vi "Process Workflow Range.vi"(8 "Parts":map{string, cluster{"Min":i64, "Max":i64}}(c390), 9 "Current Workflow":string="in", 10 "Workflow Map":map{string, string[]}(c390), 11 "Count In":i64) -> (3 "Count Out":i64)   [LabVIEW 2021]
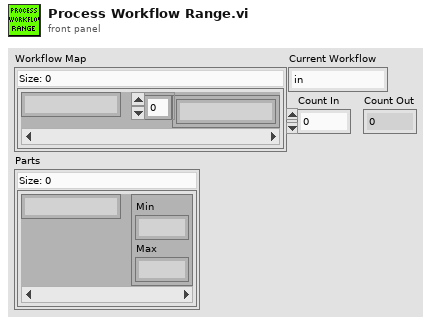
[diagram p1: front panel]
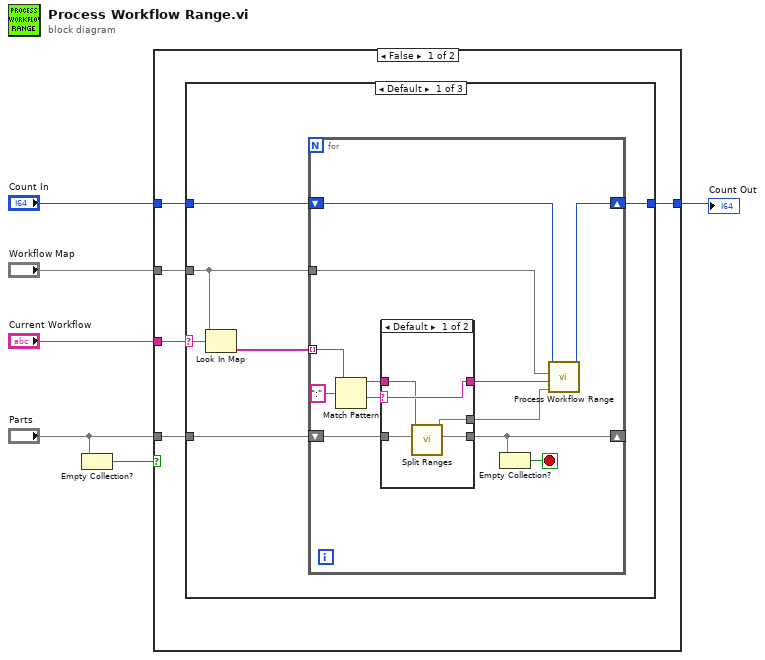
[diagram p0: block diagram]
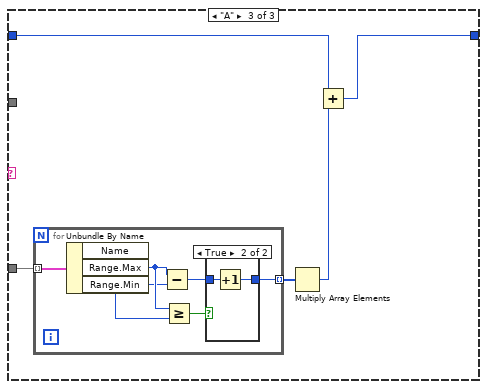
[diagram p4: hidden frame]
diagram:
  n1 = Empty Collection?(1:"Parts") -> (0:w1:bool)
  n2 = case shown="False" w1 {
    tunnel: "Current Workflow" -> [w11 _]
    tunnel: "Workflow Map" -> [w10 _]
    tunnel: "Count In" -> [w9 w51]
    tunnel: [w8 w51] -> w3
    tunnel: "Parts" -> [w7 _]
    frame False {
      n3 = case shown="Default" w11 {
        selector: w11 -> [w17 _ _]
        tunnel: w10 -> [w12 _ _]
        tunnel: w9 -> [w16 w37 w39]
        tunnel: [w15 w37 w38] -> w8
        tunnel: w7 -> [w13 _ w42]
        frame Default {
          n4 = Look In Map(map=w12, key=w17) -> (value=w14:string[])  [unwired: 1 in, 1 out]
          n5 = for {
            shift-right: [w21] -> w15
            shift-left: w16 -> [w22]
            tunnel: w14 -> [w26] mode=indexing
            tunnel: w12 -> [w23]
            shift-right: [w19] -> _
            shift-left: w13 -> [w25]
            stop <- w18 stop-if-true
            n6 = Match Pattern(string=w26, regular expression=":") -> (before substring=w27:string, after substring=w28:string)  [unwired: 1 in, 2 out]
            n7 = case shown="Default" w28 {
              selector: w28 -> [w34 _]
              tunnel: w27 -> [w30 w36]
              tunnel: [w34 w36] -> w24
              tunnel: w25 -> [w31 w35]
              tunnel: [w32 _] -> w19
              tunnel: [w33 w35] -> w20
              frame Default {
                n8 = call "Split Ranges.vi"("Parts In"=w31, "Expression"=w30) -> ("Parts Out Fail"=w32:map{string, cluster{"Min":i64, "Max":i64}}, "Parts Out Pass"=w33:map{string, cluster{"Min":i64, "Max":i64}})  [unwired: 8 in]
              }
              frame "" {
              }
            }
            n9 = Empty Collection?(1:w19) -> (0:w18:bool)
            n10 = call "Process Workflow Range.vi"("Parts"=w20, "Current Workflow"=w24, "Workflow Map"=w23, "Count In"=w22) -> ("Count Out"=w21:i64)  [unwired: 7 in]
          }
        }
        frame "R" {
        }
        frame "A" {
          n11 = for {
            tunnel: w42 -> [w48] mode=indexing
            tunnel: [w46] -> w41 mode=indexing
            n12 = Unbundle By Name(w48) -> ("Range.Max"=w45:i64, "Range.Min"=w44:i64)  [unwired: 1 out]
            n13 = Subtract(x=w45, y=w44) -> (x-y=w47:i64)
            n14 = Greater Or Equal?(x=w45, y=w44) -> (x >= y?=w43:bool)
            n15 = case shown="True" w43 {
              tunnel: w47 -> [_ w50]
              tunnel: [_ w49] -> w46
              frame False {
              }
              frame True {
                n16 = Increment(x=w50) -> (x+1=w49:i64)
              }
            }
          }
          n17 = Multiply Array Elements(1:w41) -> (0:w40:i64)
          n18 = Add(x=w39, y=w40) -> (x+y=w38:i64)
        }
      }
    }
    frame True {
    }
  }
  "Count Out" <- w3
